vi "Config - Read.vi"(8 "error in (no error)":errorcluster, 11 "View Model":T1) -> (0 "error out":errorcluster, 3 "View Model":T1)   [LabVIEW 2017]
doc: "Reads the Configuration DB and store the data into DVR\n[Covers: SD3]"
uses:
  Model/Controls/View Model.ctl
  Model/Controls/Shared Model.ctl
  Error Handler/Controls/Error Model.ctl
  Error Handler/Controls/Error Message.ctl
  Error Handler/Controls/Error Type.ctl
  Controls/Config Model.ctl
  Controls/Config DB Message.ctl
  Controls/Config DB Command.ctl
  Controls/Config DB Overhead.ctl
  Controls/Config DB Record1.ctl
  Controls/Config DB Record2.ctl
  Controller/Controls/Controller Wash Step.ctl
  Views/Vehicle Position Simulation View/Controls/Vehicle - Position.ctl
  Controller/Controls/Controller Model.ctl
  Controller/Controls/Controller Overhead.ctl
  Controller/Controls/Controller State.ctl
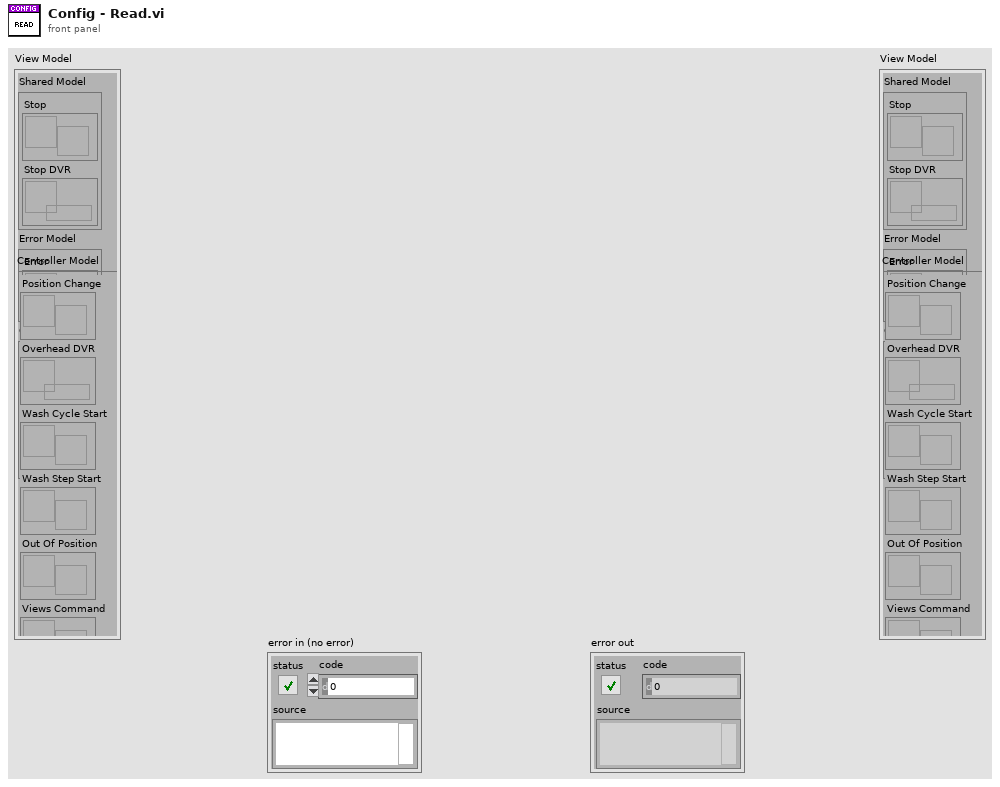
[diagram p1: front panel]
types:
  T1 = typedef "View Model.ctl" = cluster{"Shared Model":T2, "Error Model":T3, "Config Model":T4, "Controller Model":T5}
  T2 = typedef "Shared Model.ctl" = cluster{"Stop":refnum<user-event>, "Stop DVR":refnum<data-value>}
  T3 = typedef "Error Model.ctl" = cluster{"Error":refnum<user-event>}
  T4 = typedef "Config Model.ctl" = cluster{"Config":refnum<user-event>, "Config DVR":refnum<data-value>}
  T5 = typedef "Controller Model.ctl" = cluster{"Position Change":refnum<user-event>, "Overhead DVR":refnum<data-value>, "Wash Cycle Start":refnum<user-event>, "Wash Step Start":refnum<user-event>, "Out Of Position":refnum<user-event>, "Views Command":refnum<user-event>}
  T6 = typedef "Config DB Record1.ctl" = cluster{"Wash Step":string, "Station":string, "Step Duration":u32}
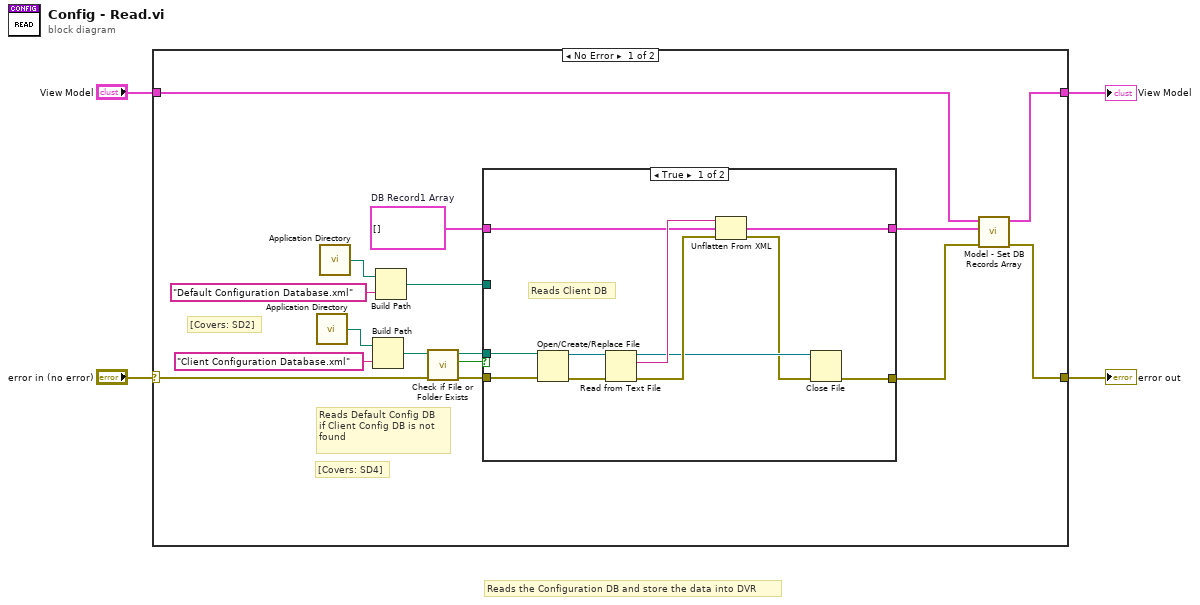
[diagram p0: block diagram]
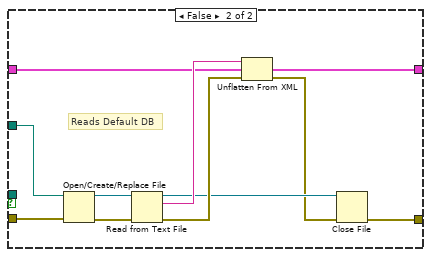
[diagram p2: hidden frame]
diagram:
  # "Reads the Configuration DB and store the data into DVR"
  n1 = case shown="No Error" "error in (no error)" {
    selector: "error in (no error)" -> [w15 w43]
    tunnel: "View Model" -> [w9 w44]
    tunnel: [w7 w43] -> w2
    tunnel: [w8 w44] -> w1
    frame No Error {
      w10 = T6[] []  # DB Record1 Array
      # "[Covers: SD4]"
      # "Reads Default Config DB\nif Client Config DB is not\nfound"
      # "[Covers: SD2]"
      n2 = call <vilib>:"Application Directory.vi"() -> ("Application Directory"=w20:path)
      n3 = call <vilib>:"Application Directory.vi"() -> ("Application Directory"=w17:path)
      n4 = Build Path(base path=w20, name or relative path="Client Configuration Database.xml") -> (appended path=w16:path)
      n5 = Build Path(base path=w17, name or relative path="Default Configuration Database.xml") -> (appended path=w12:path)
      n6 = call <vilib>:"Check if File or Folder Exists.vi"("error in (no error)"=w15, "path"=w16) -> ("error out"=w11:errorcluster, "file or folder exists?"=w14:bool, "dup path"=w13:path)  [unwired: 7 in]
      n7 = case shown="True" w14 {
        tunnel: w13 -> [w31 _]
        tunnel: w12 -> [_ w33]
        tunnel: w11 -> [w30 w42]
        tunnel: w10 -> [w26 w38]
        tunnel: [w22 w34] -> w6
        tunnel: [w21 w32] -> w5
        frame True {
          # "Reads Client DB"
          n8 = Open/Create/Replace File(file path (use dialog)=w31, error in=w30) -> (refnum out=w29:refnum<file>, error out=w28:errorcluster)  [unwired: 4 in, 1 out]
          n9 = Read from Text File(file (use dialog)=w29, error in=w28) -> (refnum out=w24:refnum<file>, text=w27:string, error out=w25:errorcluster)  [unwired: 2 in, 1 out]
          n10 = Unflatten From XML(xml string=w27, type=w26, error in (no error)=w25) -> (value=w21:T6[], error out=w23:errorcluster)
          n11 = Close File(refnum=w24, error in=w23) -> (error out=w22:errorcluster)  [unwired: 1 out]
        }
        frame False {
          # "Reads Default DB"
          n12 = Open/Create/Replace File(file path (use dialog)=w33, error in=w42) -> (refnum out=w41:refnum<file>, error out=w40:errorcluster)  [unwired: 4 in, 1 out]
          n13 = Read from Text File(file (use dialog)=w41, error in=w40) -> (refnum out=w36:refnum<file>, text=w39:string, error out=w37:errorcluster)  [unwired: 2 in, 1 out]
          n14 = Unflatten From XML(xml string=w39, type=w38, error in (no error)=w37) -> (value=w32:T6[], error out=w35:errorcluster)
          n15 = Close File(refnum=w36, error in=w35) -> (error out=w34:errorcluster)  [unwired: 1 out]
        }
      }
      n16 = call "Model - Set DB Records Array.vi"("error in (no error)"=w6, "DB Records Array"=w5, "View Model"=w9) -> ("error out"=w7:errorcluster, "View Model"=w8:T1)  [unwired: 7 in]
    }
    frame Error {
    }
  }
  "View Model" <- w1
  "error out" <- w2
